vi "VCS Deactivate Position Compare.vi"(8 "error in (no error)":errorcluster, 9 "digitalOutputNumber":u16, 11 "axis in":cluster{"keyHandle":u32, "nodeId":u16}={"keyHandle"=0, "nodeId"=1}) -> (0 "error out":errorcluster, 3 "axis out":cluster{"keyHandle":u32, "nodeId":u16}={"keyHandle"=0, "nodeId"=1})   [LabVIEW 2010]
doc: "<B>VCS_DeactivatePositionCompare</B> disables the output to position compare method."
uses:
  Resources/EposCmd.dll
  Resources/EposCmd64.dll
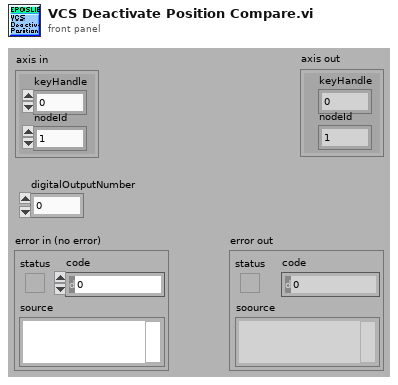
[diagram p1: front panel]
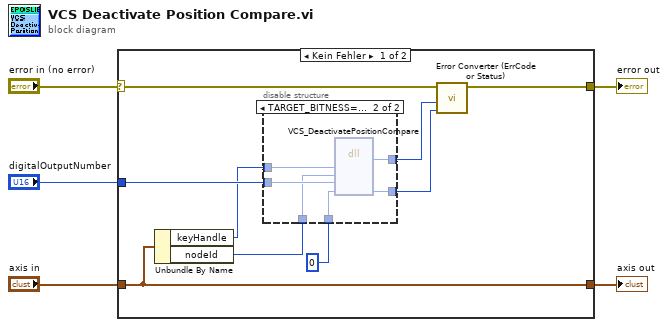
[diagram p0: block diagram]
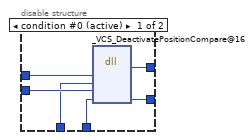
[diagram p2: hidden frame]
diagram:
  n1 = case shown="Kein Fehler" "error in (no error)" {
    selector: "error in (no error)" -> [w12 w27]
    tunnel: "axis in" -> [w14 w28]
    tunnel: [w14 w28] -> w4
    tunnel: [w13 w27] -> w3
    tunnel: "digitalOutputNumber" -> [w11 _]
    frame No Error {
      n2 = Unbundle By Name(w14) -> ("keyHandle"=w7:u32, "nodeId"=w6:u16)
      n3 = disable-structure shown="TARGET_BITNESS==64" {
        disable-tunnel: w11 -> [w20 w26]
        disable-tunnel: u32 0 ("pErrorCode") -> [w19 w25]
        disable-tunnel: [w18 w24] -> w9
        disable-tunnel: [w17 w23] -> w8
        disable-tunnel: w7 -> [w16 w22]
        disable-tunnel: w6 -> [w15 w21]
        frame condition #0 (active) {
          n4 = dll-call lib="C:/Sources/LabView/maxon EPOS/Resources/EposCmd.*" fn="_VCS_DeactivatePositionCompare@16"("KeyHandle"=w16, "NodeId"=w15, "DigitalOutputNumber"=w20, "pErrorCode"=w19) -> (w17:i32, "pErrorCode"=w18:u32)  [unwired: 6 in, 2 out]
        }
        frame condition #1 {
          n5 = dll-call lib="C:/setup/Resources/EposCmd64.*" fn="VCS_DeactivatePositionCompare" ("EposCmd.dll:_VCS_DeactivatePositionCompare@16")("KeyHandle"=w22, "NodeId"=w21, "DigitalOutputNumber"=w26, "pErrorCode"=w25) -> ("Rückgabetyp"=w23:i32, "pErrorCode"=w24:u32)  [unwired: 6 in, 2 out]
        }
      }
      n6 = call "Error Converter (ErrCode or Status).vi"("error code"=w9, "return type"=w8, "error in (no error)"=w12) -> ("error out"=w13:errorcluster)  [unwired: 7 in]
    }
    frame Error {
    }
  }
  "error out" <- w3
  "axis out" <- w4
